vi "Find Available COM Ports.vi"() -> (2 "Array":string[](array[string]))   [LabVIEW 2025]
uses:
  <vilib>/Instr/_visa.llb/VISA Find Search Mode.ctl
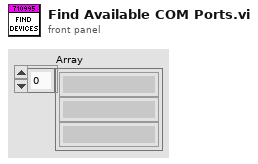
[diagram p1: front panel]
types:
  T1 = typedef "VISA Find Search Mode.ctl" = u32
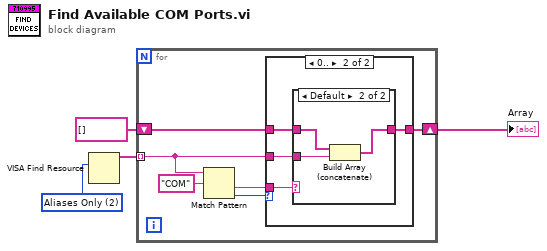
[diagram p0: block diagram]
diagram:
  w4 = T1 2 items=["Canonical Names Only"=0, "Aliases Only"=2, "Include Matching Aliases"=3, "Include All Aliases"=4] ("Search Mode")
  n1 = VISA Find Resource(10:w4) -> (3:w3:string[])  [unwired: 2 in, 2 out]
  n2 = for {
    tunnel: w3 -> [w8] mode=indexing
    shift-right: [w7] -> w1
    shift-left: string[] [] -> [w6]
    n3 = Match Pattern(string=w8, regular expression="COM") -> (after substring=w5:string, offset past match=w9:i32)  [unwired: 1 in, 2 out]
    n4 = case shown="0.." w9 {
      tunnel: w8 -> [_ w15]
      tunnel: [w11 w14] -> w7
      tunnel: w6 -> [w11 w13]
      tunnel: w5 -> [_ w12]
      frame -1, Default {
      }
      frame 0.. {
        n5 = case shown="Default" w12 {
          tunnel: w15 -> [_ w19]
          tunnel: [w16 w18] -> w14
          tunnel: w13 -> [w16 w17]
          frame "3" {
          }
          frame Default {
            n6 = Build Array (concatenate)(w17, w19) -> (w18:string[])
          }
        }
      }
    }
  }
  "Array" <- w1
